vi "Find Charge Transitions.vi"(6 "Dielectric Constant":dbl=11.0, 8 "Volume (A³)":dbl=7795.605843681768, 9 "Markov-Payne Corrections":bool, 10 "VBM":dbl=1.8, 11 "Defect Data":T2={"Defect Details"={"Defect Name"="", "Site Density"=0.0, "Reference Pure Structure Energy"=-358.247, "N (Cd,Ideal - Cd,Defect)"=0, "N (Te,ideal - Te,defect)"=0}, "Charges and Energies"=[]}) -> (3 "Transitions":T1(array[cluster]))   [LabVIEW 2010]
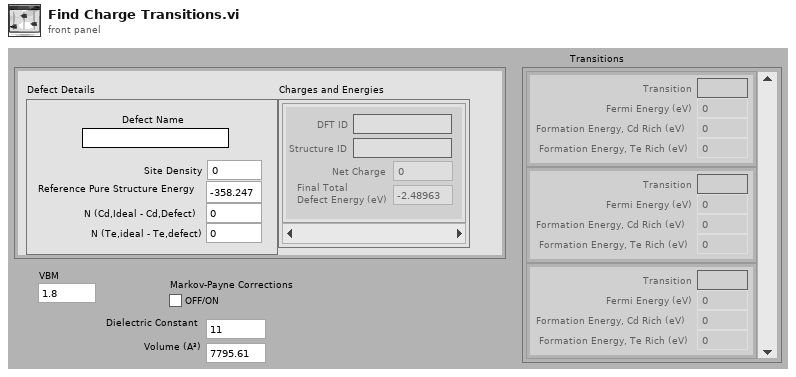
[diagram p1: front panel]
types:
  T1 = cluster{"Transition":string, "Fermi Energy (eV)":dbl, "Formation Energy, Cd Rich (eV)":dbl, "Formation Energy, Te Rich (eV)":dbl}[]
  T2 = cluster{"Defect Details":cluster{"Defect Name":string, "Site Density":dbl, "Reference Pure Structure Energy":dbl, "N (Cd,Ideal - Cd,Defect)":i32, "N (Te,ideal - Te,defect)":i32}, "Charges and Energies":cluster{"DFT ID":string, "Structure ID":string, "Net Charge":i32, "Final Total \nDefect Energy (eV)":dbl}[]}
  T3 = cluster{"Defect Name":string, "Site Density":dbl, "Reference Pure Structure Energy":dbl, "N (Cd,Ideal - Cd,Defect)":i32, "N (Te,ideal - Te,defect)":i32}
  T4 = cluster{"DFT ID":string, "Structure ID":string, "Net Charge":i32, "Final Total \nDefect Energy (eV)":dbl}[]
  T5 = cluster{"DFT ID":string, "Structure ID":string, "Net Charge":i32, "Final Total \nDefect Energy (eV)":dbl}
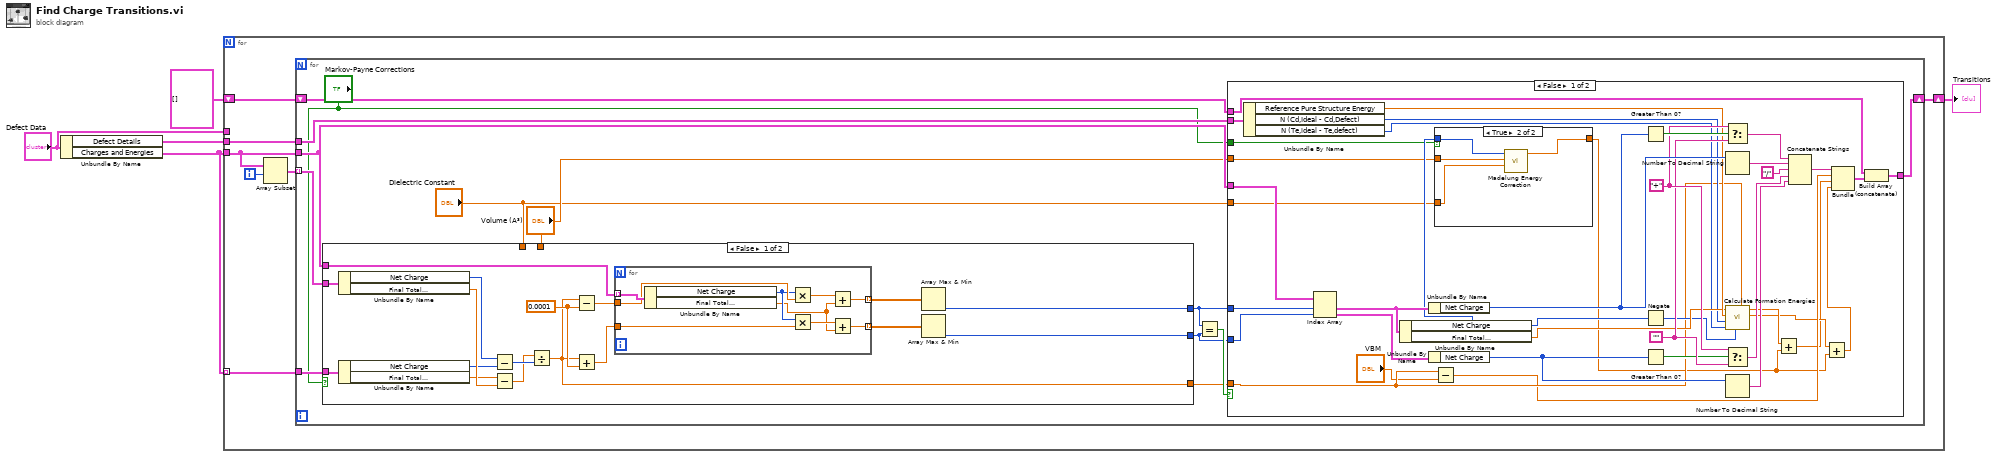
[diagram p0: block diagram]
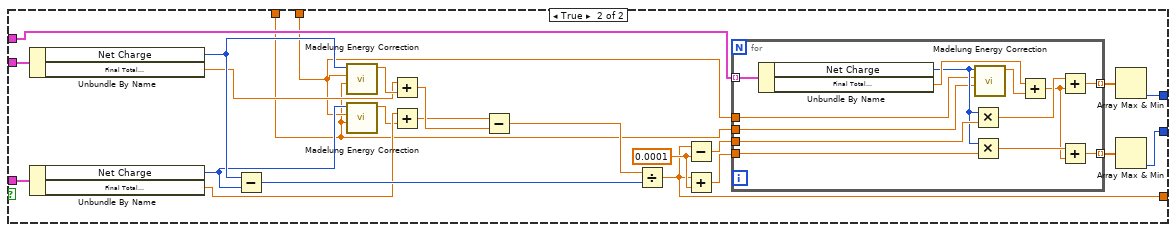
[diagram p2: hidden frame]
diagram:
  n1 = Unbundle By Name("Defect Data") -> ("Defect Details"=w3:T3, "Charges and Energies"=w5:T4)
  n2 = for {
    tunnel: w5 -> [w12] mode=indexing
    tunnel: w5 -> [w9]
    shift-right: [w8] -> w4
    shift-left: T1 [] ("Transitions 2") -> [w7]
    tunnel: w3 -> [w6]
    tunnel: "Defect Data" -> [_]
    i -> [w11]
    n3 = Array Subset(array=w9, index=w11) -> (w10:T4)  [unwired: 1 in]
    n4 = for {
      tunnel: w12 -> [w16]
      tunnel: w10 -> [w17] mode=indexing
      tunnel: w9 -> [w24]
      shift-right: [w20] -> w8
      shift-left: w7 -> [w19]
      tunnel: w6 -> [w18]
      n5 = case shown="False" "Markov-Payne Corrections" {
        tunnel: w24 -> [w35 w67]
        tunnel: [w34 w66] -> w23
        tunnel: [w33 w65] -> w22
        tunnel: [w32 w64] -> w21
        tunnel: w17 -> [w31 w63]
        tunnel: w16 -> [w28 w62]
        tunnel: "Volume (A³)" -> [_ w53]
        tunnel: "Dielectric Constant" -> [_ w52]
        frame False {
          w40 = 0.0001 ("y")
          n6 = Unbundle By Name(w31) -> ("Net Charge"=w30:i32, "Final Total \nDefect Energy (eV)"=w29:dbl)
          n7 = Unbundle By Name(w28) -> ("Net Charge"=w27:i32, "Final Total \nDefect Energy (eV)"=w26:dbl)
          n8 = Subtract(x=w30, y=w27) -> (x-y=w42:i32)
          n9 = Subtract(x=w26, y=w29) -> (x-y=w41:dbl)
          n10 = Divide(x=w41, y=w42) -> (x/y=w32:dbl)
          n11 = Subtract(x=w32, y=w40) -> (x-y=w39:dbl)
          n12 = Add(x=w32, y=w40) -> (x+y=w38:dbl)
          n13 = for {
            tunnel: w35 -> [w51] mode=indexing
            tunnel: w39 -> [w50]
            tunnel: w38 -> [w47]
            tunnel: [w46] -> w37 mode=indexing
            tunnel: [w45] -> w36 mode=indexing
            n14 = Unbundle By Name(w51) -> ("Net Charge"=w44:i32, "Final Total \nDefect Energy (eV)"=w43:dbl)
            n15 = Multiply(x=w44, y=w50) -> (x*y=w49:dbl)
            n16 = Multiply(x=w44, y=w47) -> (x*y=w48:dbl)
            n17 = Add(x=w49, y=w43) -> (x+y=w46:dbl)
            n18 = Add(x=w48, y=w43) -> (x+y=w45:dbl)
          }
          n19 = Array Max & Min(array=w37) -> (min index (indices)=w34:i32)  [unwired: 3 out]
          n20 = Array Max & Min(array=w36) -> (min index (indices)=w33:i32)  [unwired: 3 out]
        }
        frame True {
          w72 = 0.0001 ("y")
          n21 = Unbundle By Name(w63) -> ("Net Charge"=w61:i32, "Final Total \nDefect Energy (eV)"=w59:dbl)
          n22 = Unbundle By Name(w62) -> ("Net Charge"=w57:i32, "Final Total \nDefect Energy (eV)"=w56:dbl)
          n23 = Subtract(x=w61, y=w57) -> (x-y=w74:i32)
          n24 = call "Madelung Energy Correction.vi"("Dielectric Constant"=w52, "Volume (A³)"=w53, "Net Charge"=w61) -> ("1st Order correction (eV)"=w60:dbl)  [unwired: 7 in, 1 out]
          n25 = call "Madelung Energy Correction.vi"("Dielectric Constant"=w52, "Volume (A³)"=w53, "Net Charge"=w57) -> ("1st Order correction (eV)"=w54:dbl)  [unwired: 7 in, 1 out]
          n26 = Add(x=w59, y=w60) -> (x+y=w58:dbl)
          n27 = Add(x=w56, y=w54) -> (x+y=w55:dbl)
          n28 = Subtract(x=w55, y=w58) -> (x-y=w73:dbl)
          n29 = Divide(x=w73, y=w74) -> (x/y=w64:dbl)
          n30 = Subtract(x=w64, y=w72) -> (x-y=w71:dbl)
          n31 = Add(x=w64, y=w72) -> (x+y=w70:dbl)
          n32 = for {
            tunnel: w67 -> [w87] mode=indexing
            tunnel: w71 -> [w86]
            tunnel: w70 -> [w83]
            tunnel: [w82] -> w69 mode=indexing
            tunnel: [w81] -> w68 mode=indexing
            tunnel: w53 -> [w76]
            tunnel: w52 -> [w75]
            n33 = Unbundle By Name(w87) -> ("Net Charge"=w77:i32, "Final Total \nDefect Energy (eV)"=w80:dbl)
            n34 = Multiply(x=w77, y=w86) -> (x*y=w85:dbl)
            n35 = Multiply(x=w77, y=w83) -> (x*y=w84:dbl)
            n36 = call "Madelung Energy Correction.vi"("Dielectric Constant"=w75, "Volume (A³)"=w76, "Net Charge"=w77) -> ("1st Order correction (eV)"=w78:dbl)  [unwired: 7 in, 1 out]
            n37 = Add(x=w80, y=w78) -> (x+y=w79:dbl)
            n38 = Add(x=w85, y=w79) -> (x+y=w82:dbl)
            n39 = Add(x=w84, y=w79) -> (x+y=w81:dbl)
          }
          n40 = Array Max & Min(array=w69) -> (min index (indices)=w66:i32)  [unwired: 3 out]
          n41 = Array Max & Min(array=w68) -> (min index (indices)=w65:i32)  [unwired: 3 out]
        }
      }
      n42 = Equal?(x=w23, y=w22) -> (x = y?=w25:bool)
      n43 = case shown="False" w25 {
        tunnel: w24 -> [w125 _]
        tunnel: w23 -> [w124 _]
        tunnel: w22 -> [w123 _]
        tunnel: w21 -> [w99 _]
        tunnel: [w107 w130] -> w20
        tunnel: w19 -> [w109 w130]
        tunnel: w18 -> [w106 _]
        tunnel: "Markov-Payne Corrections" -> [w90 _]
        tunnel: "Volume (A³)" -> [w89 _]
        tunnel: "Dielectric Constant" -> [w88 _]
        frame False {
          w114 = ""
          w115 = "+"
          n44 = Unbundle By Name(w106) -> ("Reference Pure Structure Energy"=w105:dbl, "N (Cd,Ideal - Cd,Defect)"=w102:i32, "N (Te,ideal - Te,defect)"=w101:i32)
          n45 = Index Array(array=w125, index #1=w124, index #2=w123) -> (element #1=w100:T5, element #2=w122:T5)
          n46 = Unbundle By Name(w100) -> ("Net Charge"=w96:i32, "Final Total \nDefect Energy (eV)"=w104:dbl)
          n47 = Unbundle By Name(w100) -> ("Net Charge"=w121:i32)
          n48 = Unbundle By Name(w122) -> ("Net Charge"=w120:i32)
          n49 = case shown="True" w90 {
            tunnel: w96 -> [_ w129]
            tunnel: [_ w128] -> w93
            tunnel: w89 -> [_ w127]
            tunnel: w88 -> [_ w126]
            frame False {
            }
            frame True {
              n50 = call "Madelung Energy Correction.vi"("Dielectric Constant"=w126, "Volume (A³)"=w127, "Net Charge"=w129) -> ("1st Order correction (eV)"=w128:dbl)  [unwired: 7 in, 1 out]
            }
          }
          n51 = Subtract(x=w99, y="VBM") -> (x-y=w97:dbl)
          n52 = Greater Than 0?(x=w121) -> (x > 0?=w119:bool)
          n53 = Negate(x=w96) -> (-x=w103:i32)
          n54 = Greater Than 0?(x=w120) -> (x > 0?=w113:bool)
          n55 = Select(t=w115, s=w119, f=w114) -> (s? t:f=w118:string)
          n56 = Number To Decimal String(number=w121) -> (decimal integer string=w117:string)  [unwired: 1 in]
          n57 = call "Calculate Formation Energies.vi"("Fermi (electron) energy (eV)"=w99, "# Extra Electrons"=w103, "N (Te,ideal - Te,defect)"=w101, "N (Cd,Ideal - Cd,Defect)"=w102, "Reference Pure Structure Energy"=w105, "Final Total Defect Energy (eV)"=w104) -> ("Formation Energy (Te-Rich)"=w94:dbl, "Formation Energy (Cd-Rich)"=w95:dbl)  [unwired: 4 in]
          n58 = Select(t=w115, s=w113, f=w114) -> (s? t:f=w112:string)
          n59 = Number To Decimal String(number=w120) -> (decimal integer string=w111:string)  [unwired: 1 in]
          n60 = Add(x=w95, y=w93) -> (x+y=w92:dbl)
          n61 = Concatenate Strings(w118, w117, "/" ("string"), w112, w111) -> (w110:string)
          n62 = Add(x=w94, y=w93) -> (x+y=w91:dbl)
          n63 = Bundle(w110, w97, w92, w91) -> (w108:cluster{string, dbl, dbl, dbl})  [unwired: 1 in]
          n64 = Build Array (concatenate)(w109, w108) -> (w107:T1)
        }
        frame True {
        }
      }
    }
  }
  "Transitions" <- w4
